vi "Rx Message to Transfer Handle.vi"(8 "error in":errorcluster, 9 "message":T2={"name"="", "message type"="BC to RT", "endpoint Tx"={"terminal address"=0, "subaddress"=0}, "endpoint Rx"={"terminal address"=0, "subaddress"=0}, "create timestamp channel"=FALSE, "mode code"=0, "number of words"=0, "parameters"=[]}, 10 "remote terminal handles":u64[](array[numeric]), 11 "bus controller handle":u64) -> (0 "error out":errorcluster, 2 "valid?":bool, 3 "Rx read info":T1)   [LabVIEW 2020, in "Ballard MIL-STD-1553 Engine.lvlib" / "Custom Device.lvlib"]
uses:
  Custom Device.lvlib
  Shared/Message Definition.ctl
  Shared/Message Type.ctl
  Shared/Terminal Endpoint.ctl
  Shared/Address.ctl
  Shared/Parameter Definition.ctl
  Shared/Rx Read Info.ctl
  <instrlib>/BTI1553Lib/Public/Controls/1553 RT Transfer Type.ctl
  <instrlib>/BTI1553Lib/Public/Controls/1553 Transfer Direction.ctl
  <instrlib>/BTI1553Lib/Private/RT/Configure/Get RT Xfer Handle.vi
  <instrlib>/BTI1553Lib/BTI1553LV.lvlib
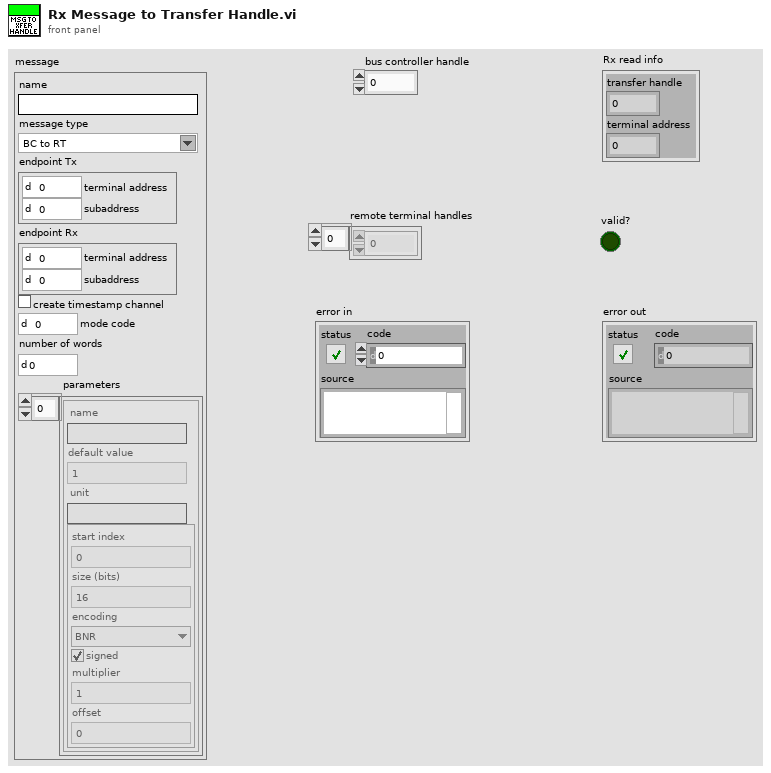
[diagram p1: front panel]
types:
  T1 = typedef "Rx Read Info.ctl" = cluster{"transfer handle":u64, "terminal address":u16}
  T2 = typedef "Message Definition.ctl" = cluster{"name":string, "message type":T3, "endpoint Tx":T4, "endpoint Rx":T4, "create timestamp channel":bool, "mode code":u16, "number of words":u16, "parameters":cluster{"name":string, "default value":dbl, "unit":string, "parameter definition":T6}[]}
  T3 = typedef "Message Type.ctl" = string
  T4 = typedef "Terminal Endpoint.ctl" = cluster{"terminal address":T5, "subaddress":T5}
  T5 = typedef "Address.ctl" = u16
  T6 = typedef "Parameter Definition.ctl" = cluster{"start index":i32, "size (bits)":i32, "encoding":enum16{"BNR", "BCD", "Discrete"}, "signed":bool, "multiplier":dbl, "offset":dbl}
  T7 = typedef "BTI1553LV.lvlib/1553 Transfer Direction.ctl" = u32
  T8 = typedef "BTI1553LV.lvlib/1553 RT Transfer Type.ctl" = u32
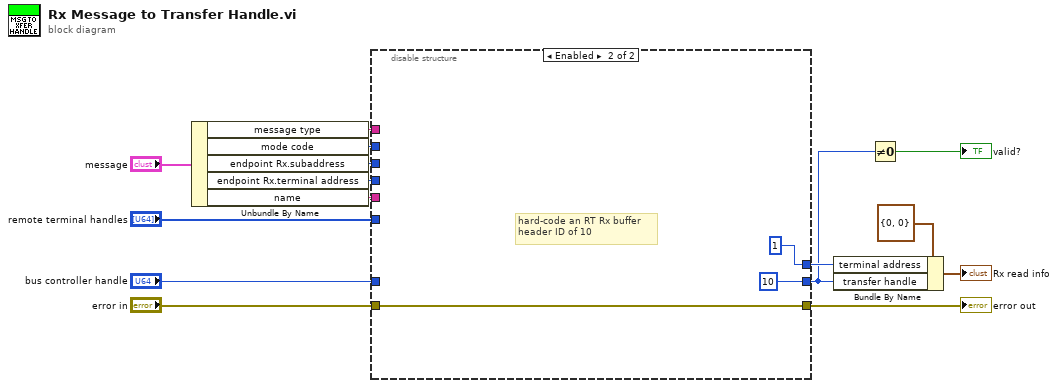
[diagram p0: block diagram]
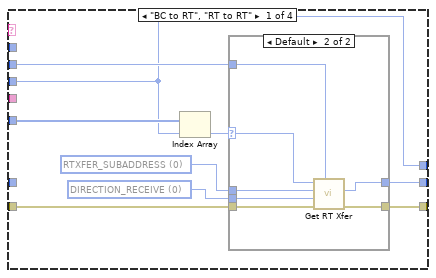
[diagram p3: hidden frame]
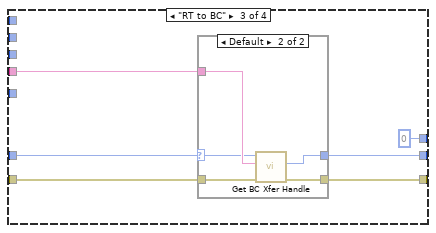
[diagram p5: hidden frame]
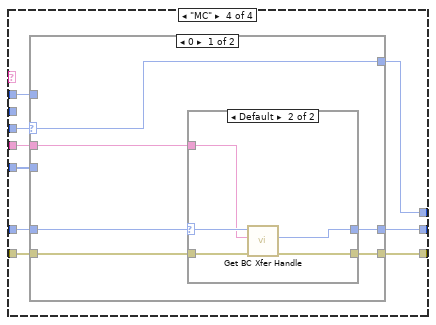
[diagram p7: hidden frame]
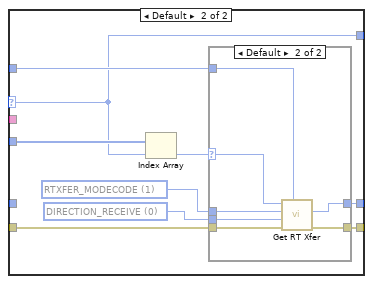
[diagram p9: hidden frame]
diagram:
  n1 = Unbundle By Name("message") -> ("message type"=w6:T3, "mode code"=w12:u16, "endpoint Rx.subaddress"=w15:T5, "endpoint Rx.terminal address"=w14:T5, "name"=w7:string)
  n2 = disable-structure shown="Enabled" {
    disable-tunnel: w15 -> [w26 _]
    disable-tunnel: w14 -> [w25 _]
    disable-tunnel: w12 -> [w24 _]
    disable-tunnel: "error in" -> [w23 w95]
    disable-tunnel: "remote terminal handles" -> [w22 _]
    disable-tunnel: [w21 w95] -> w9
    disable-tunnel: "bus controller handle" -> [w20 _]
    disable-tunnel: w7 -> [w19 _]
    disable-tunnel: w6 -> [w18 _]
    disable-tunnel: [w17 T5 1 ("terminal address")] -> w3
    disable-tunnel: [w16 u64 10 ("rt transfer handle out")] -> w1
    frame Disabled {
      n3 = case shown="Default" w18 {
        tunnel: w26 -> [w28 _ _ _]
        tunnel: w25 -> [w27 _ _ w65]
        tunnel: w24 -> [_ _ _ w61]
        tunnel: w23 -> [w35 w44 w48 w64]
        tunnel: w22 -> [w32 _ _ w62]
        tunnel: [w30 _ w50 w60] -> w16
        tunnel: [w29 w44 w47 w63] -> w21
        tunnel: w20 -> [_ _ w49 w59]
        tunnel: w19 -> [_ _ w45 w58]
        tunnel: [w27 _ T5 0 ("terminal address") w57] -> w17
        frame "BC to RT", "RT to RT" {
          w34 = T7 0 items=["DIRECTION_RECEIVE", "DIRECTION_TRANSMIT"] ("transfer direction")
          w33 = T8 0 items=["RTXFER_SUBADDRESS", "RTXFER_MODECODE"] ("transfer type")
          n4 = Index Array(array=w32, index=w27) -> (element=w31:u64)
          n5 = case shown="Default" w31 {
            selector: w31 -> [_ w40]
            tunnel: w35 -> [w36 w43]
            tunnel: w34 -> [_ w42]
            tunnel: w33 -> [_ w41]
            tunnel: [_ w39] -> w30
            tunnel: [w36 w38] -> w29
            tunnel: w28 -> [_ w37]
            frame 0, -1 {
            }
            frame Default {
              n6 = call-poly <instrlib>:"Get RT Xfer.vi"("transfer sa number or mc number"=w37, "error in (no error)"=w43, "transfer direction"=w42, "transfer type"=w41, "remote terminal handle in"=w40) -> ("error out"=w38:errorcluster, "rt transfer handle out"=w39:u64)  [unwired: 4 in, 1 out]
            }
          }
        }
        frame Default {
        }
        frame "RT to BC" {
          n7 = case shown="Default" w49 {
            selector: w49 -> [_ w54]
            tunnel: [_ w56] -> w50
            tunnel: w45 -> [_ w55]
            tunnel: w48 -> [w51 w53]
            tunnel: [w51 w52] -> w47
            frame 0, -1 {
            }
            frame Default {
              n8 = call <instrlib>:"Get BC Xfer Handle.vi"("error in (no error)"=w53, "bc transfer name"=w55, "bus controller handle in"=w54) -> ("error out"=w52:errorcluster, "bc transfer handle out"=w56:u64)  [unwired: 6 in, 1 out]
            }
          }
        }
        frame "MC" {
          n9 = case shown="0" w65 {
            selector: w65 -> [w67 w78]
            tunnel: w64 -> [w71 w86]
            tunnel: [w70 w85] -> w63
            tunnel: w62 -> [_ w82]
            tunnel: w61 -> [_ w80]
            tunnel: [w68 w79] -> w60
            tunnel: w59 -> [w69 _]
            tunnel: w58 -> [w66 _]
            tunnel: [w67 w78] -> w57
            frame 0 {
              n10 = case shown="Default" w69 {
                selector: w69 -> [_ w75]
                tunnel: w71 -> [w72 w77]
                tunnel: [w72 w76] -> w70
                tunnel: w66 -> [_ w73]
                tunnel: [_ w74] -> w68
                frame 0, -1 {
                }
                frame Default {
                  n11 = call <instrlib>:"Get BC Xfer Handle.vi"("error in (no error)"=w77, "bc transfer name"=w73, "bus controller handle in"=w75) -> ("error out"=w76:errorcluster, "bc transfer handle out"=w74:u64)  [unwired: 6 in, 1 out]
                }
              }
            }
            frame Default {
              w83 = T8 1 items=["RTXFER_SUBADDRESS", "RTXFER_MODECODE"] ("transfer type")
              w84 = T7 0 items=["DIRECTION_RECEIVE", "DIRECTION_TRANSMIT"] ("transfer direction")
              n12 = Index Array(array=w82, index=w78) -> (element=w81:u64)
              n13 = case shown="Default" w81 {
                selector: w81 -> [_ w90]
                tunnel: w86 -> [w87 w94]
                tunnel: [w87 w93] -> w85
                tunnel: w84 -> [_ w92]
                tunnel: w83 -> [_ w91]
                tunnel: w80 -> [_ w89]
                tunnel: [_ w88] -> w79
                frame 0, -1 {
                }
                frame Default {
                  n14 = call-poly <instrlib>:"Get RT Xfer.vi"("transfer sa number or mc number"=w89, "error in (no error)"=w94, "transfer direction"=w92, "transfer type"=w91, "remote terminal handle in"=w90) -> ("error out"=w93:errorcluster, "rt transfer handle out"=w88:u64)  [unwired: 4 in, 1 out]
                }
              }
            }
          }
        }
      }
    }
    frame Enabled {
      # "hard-code an RT Rx buffer\nheader ID of 10"
    }
  }
  "error out" <- w9
  n15 = Bundle By Name(cluster=T1 {"transfer handle"=0, "terminal address"=0} ("Rx read info"), "terminal address"=w3, "transfer handle"=w1) -> (→"Rx read info":T1)
  n16 = Not Equal To 0?(x=w1) -> (x != 0?=→"valid?":bool)
